vi "onExecuteJob.vi"(8 "error in (no error)":errorcluster, 10 "stdin":string, 11 "Job.SingleFileCopy in":refnum<class "Job.SingleFileCopy.lvclass">) -> (0 "error out":errorcluster, 1 "exception":i32, 2 "stdout":string, 3 "Job.SingleFileCopy":refnum<class "Job.SingleFileCopy.lvclass">)   [LabVIEW 2013, in "Job.SingleFileCopy.lvclass"]
uses:
  Job.SingleFileCopy.lvclass
  FileCopy Job Configuration -- cluster.ctl
  Job.SingleFileCopy.lvclass/Job.SingleFileCopy.ctl
  <userlib>/_OpenG.lib/file/file.llb/Valid Path - Traditional__ogtk.vi
  <userlib>/_OpenG.lib/file/file.llb/File Exists - Scalar__ogtk.vi
  <userlib>/_OpenG.lib/file/file.llb/Strip Path - Traditional__ogtk.vi
  <userlib>/_OpenG.lib/file/file.llb/Build Path - Traditional__ogtk.vi
  <vilib>/LabVIEW Open Source Project/Cron Scheduler/Job/Job.lvclass
  <vilib>/addons/_JKI.lib/Serialization/JSON/JKI JSON Serialization.lvlib
panel:
  # "RUNNING A JOB"
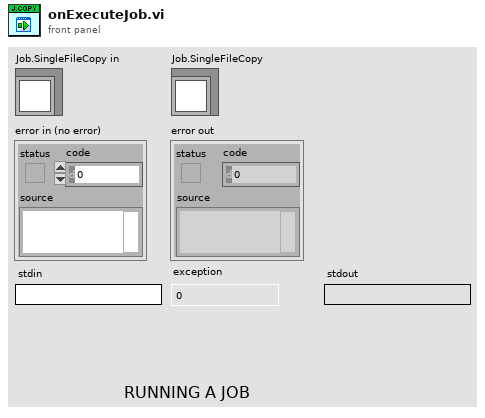
[diagram p1: front panel]
types:
  T1 = typedef "Job.SingleFileCopy.lvclass/FileCopy Job Configuration -- cluster.ctl" = cluster{"overwrite?":bool}
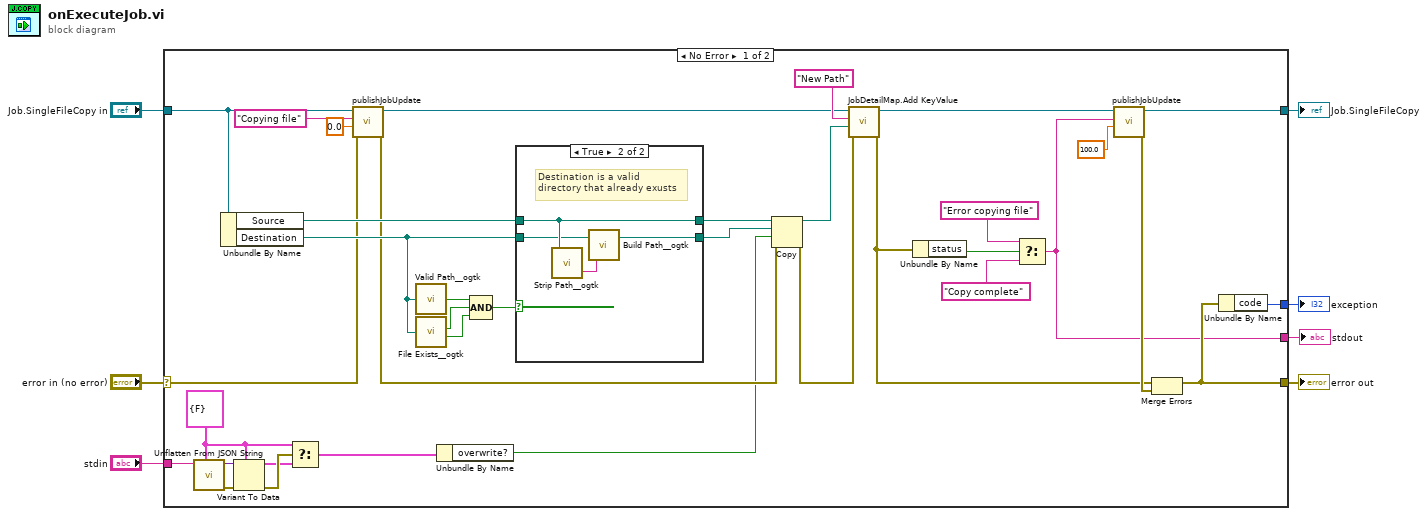
[diagram p0: block diagram]
diagram:
  n1 = case shown="No Error" "error in (no error)" {
    selector: "error in (no error)" -> [w32 w51]
    tunnel: "stdin" -> [w16 _]
    tunnel: "Job.SingleFileCopy in" -> [w36 w50]
    tunnel: [w17 w51] -> w5
    tunnel: [w29 w50] -> w3
    tunnel: [w28 _] -> w2
    tunnel: [w10 _] -> w1
    frame No Error {
      w11 = T1 {"overwrite?"=FALSE} ("FileCopy Job Config")
      n2 = call <vilib>:"Unflatten From JSON String.vi"("Type and Defaults"=w11, "JSON String"=w16) -> ("error out"=w15:errorcluster, "Variant"=w14:variant)  [unwired: 8 in]
      n3 = Unbundle By Name(w36) -> ("Source"=w38:path, "Destination"=w39:path)
      n4 = Variant To Data(error in=w15, type=w11, Variant=w14) -> (data=w12:T1, error out=w13:errorcluster)
      n5 = Select(t=w11, s=w13, f=w12) -> (s? t:f=w9:T1)
      n6 = call <vilib>:"publishJobUpdate.vi"("error in (no error)"=w32, "% Complete (NaN if unknown)"=0.0, "Status Message"="Copying file", "Job in"=w36) -> ("error out"=w24:errorcluster, "Job out"=w35:refnum<class "Job.SingleFileCopy.lvclass">)  [unwired: 6 in]
      n7 = call-poly <userlib>:"Valid Path__ogtk.vi"("path"=w39) -> ("valid"=w43:bool)
      n8 = call-poly <userlib>:"File Exists__ogtk.vi"("file path"=w39) -> ("is directory"=w42:bool, "exists"=w41:bool)  [unwired: 6 in]
      n9 = Unbundle By Name(w9) -> ("overwrite?"=w8:bool)
      n10 = Compound Arithmetic op=AND(w43, w42, w41) -> (w40:bool)
      n11 = case shown="True" w40 {
        tunnel: w39 -> [w44 w48]
        tunnel: w38 -> [w45 w49]
        tunnel: [w45 w49] -> w27
        tunnel: [w44 w46] -> w26
        frame False {
        }
        frame True {
          # "Destination is a valid\ndirectory that already exusts"
          n12 = call-poly <userlib>:"Strip Path__ogtk.vi"("path"=w49) -> ("name"=w47:string)  [unwired: 1 out]
          n13 = call-poly <userlib>:"Build Path__ogtk.vi"("name or relative path"=w47, "base path"=w48) -> ("appended path"=w46:path)
        }
      }
      n14 = Copy(8:w24, 9:w8, 10:w26, 11:w27) -> (0:w23:errorcluster, 3:w25:path)  [unwired: 1 in, 1 out]
      n15 = call <vilib>:"JobDetailMap.Add KeyValue.vi"("error in (no error)"=w23, "Value"=w25, "Key"="New Path", "Job in"=w35) -> ("error out"=w18:errorcluster, "Job out"=w30:refnum<class "Job.SingleFileCopy.lvclass">)  [unwired: 6 in]
      n16 = Unbundle By Name(w18) -> ("status"=w22:bool)
      n17 = Select(t="Error copying file" ("Status Message"), s=w22, f="Copy complete" ("Status Message")) -> (s? t:f=w10:string)
      n18 = call <vilib>:"publishJobUpdate.vi"("% Complete (NaN if unknown)"=100.0, "Status Message"=w10, "Job in"=w30) -> ("error out"=w19:errorcluster, "Job out"=w29:refnum<class "Job.SingleFileCopy.lvclass">)  [unwired: 7 in]
      n19 = Merge Errors(w18, w19) -> (w17:errorcluster)
      n20 = Unbundle By Name(w17) -> ("code"=w28:i32)
    }
    frame Error {
    }
  }
  "error out" <- w5
  "Job.SingleFileCopy" <- w3
  "exception" <- w2
  "stdout" <- w1
